vi "Get Setting - Application_Name.vi"(8 "Error In":errorcluster) -> (0 "Error Out":errorcluster, 3 "Application_Name":string)   [LabVIEW 2023, in "Error Manager.lvlib" / "Settings.lvclass"]
uses:
  Settings.lvclass
  Settings.lvclass/Settings.ctl
  Settings (class variable).vi
panel:
  # "Input\nInputs to the VI"
  # "Development\nControls or indicators that are useful for development or testing, but which are not outputs of the VI."
  # "Output\nOutputs of the VI"
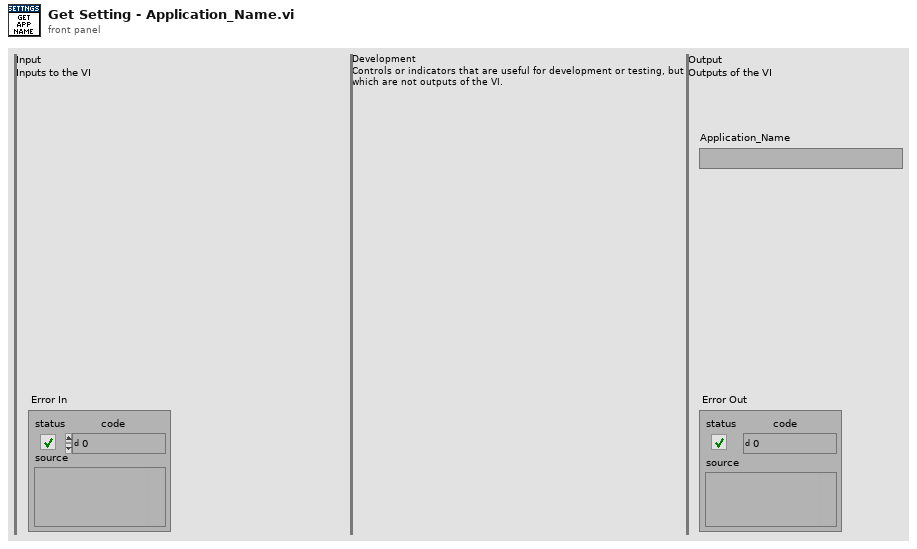
[diagram p1: front panel]
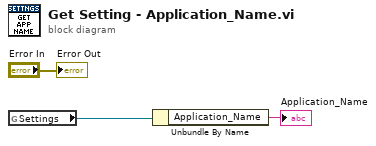
[diagram p0: block diagram]
diagram:
  n1 = global read "Settings (class variable).vi" "Settings"() -> (w1:refnum<class "Settings.lvclass">)
  n2 = Unbundle By Name(w1) -> ("Application_Name"=→"Application_Name":string)
  "Error Out" <- "Error In"
